vi "CRYReal FFT.vi"(6 "FFT size":i32=-1, 8 "Spectral Scaling":u16=1, 9 "unwrap phase (T)":bool=TRUE, 10 "Fs":dbl=1.0 format="%0.2f", 11 "Signal (V)":dbl[](array[numeric])) -> (0 "df":dbl format="%0.2f", 2 "Amp Spectrum Phase (radians)":dbl[](array[numeric]), 3 "Amp Spectrum Mag":dbl[](array[numeric]))   [LabVIEW 2013]
uses:
  <vilib>/Analysis/2dsp.llb/Real FFT.vi
  <vilib>/Analysis/NI_AALPro.lvlib
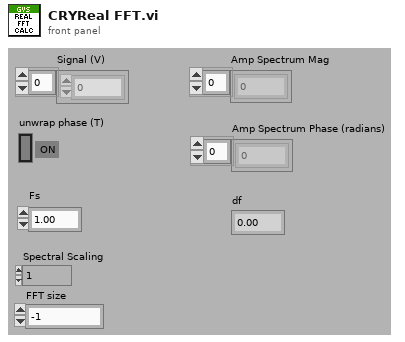
[diagram p1: front panel]
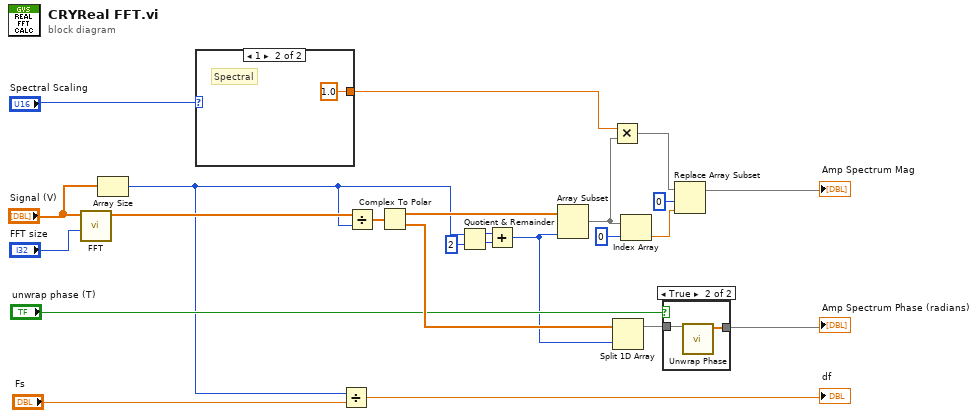
[diagram p0: block diagram]
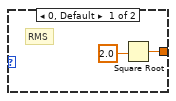
[diagram p2: hidden frame]
diagram:
  n1 = call-poly <vilib>:"FFT.vi"("FFT size"="FFT size", "X"="Signal (V)") -> ("FFT {X}"=w7:cdb[])  [unwired: 8 in, 1 out]
  n2 = Array Size(array="Signal (V)") -> (size(s)=w4:i32)
  n3 = case shown="1" "Spectral Scaling" {
    tunnel: [w25 1.0] -> w9
    frame 0, Default {
      # "RMS"
      n4 = Square Root(x=2.0) -> (sqrt(x)=w25:dbl)
    }
    frame 1 {
      # "Spectral"
    }
  }
  n5 = Divide(x=w4, y="Fs") -> (x/y=→"df":dbl)
  n6 = Divide(x=w7, y=w4) -> (x/y=w6:cdb[])
  n7 = Complex To Polar(r * e^(i*theta)=w6) -> (r=w12:dbl[], theta=w24:dbl[])
  n8 = Quotient & Remainder(x=w4, y=2) -> (x-y*floor(x/y)=w16:i32, floor(x/y)=w15:i32)
  n9 = Add(x=w16, y=w15) -> (x+y=w14:i32)
  n10 = Array Subset(array=w12, length=w14) -> (w11:dbl[])  [unwired: 1 in]
  n11 = Multiply(x=w9, y=w11) -> (x*y=w8:dbl[])
  n12 = Split 1D Array(array=w24, index=w14) -> (first subarray=w22:dbl[])  [unwired: 1 out]
  n13 = Index Array(array=w11, index=0) -> (element=w18:dbl)
  n14 = case shown="True" "unwrap phase (T)" {
    tunnel: w22 -> [w28 w30]
    tunnel: [w28 w29] -> w21
    frame False {
    }
    frame True {
      n15 = call <vilib>:"Unwrap Phase.vi"("Phase"=w30) -> ("Unwrapped Phase"=w29:dbl[])  [unwired: 9 in, 1 out]
    }
  }
  "Amp Spectrum Phase (radians)" <- w21
  n16 = Replace Array Subset(array=w8, new element=w18, index=0) -> (→"Amp Spectrum Mag":dbl[])
